vi "位置（目标角度）报文计算公式.vi"(1 "位置":dbl(slide) scale=-12.5..12.5) -> (0 "输出位置报文":string)   [LabVIEW 2023]
panel:
  out "*(类型 *) &x":string
  out "二进制":string
  out "十进制数":i32
  out "位置16进制报文":string
  out "位置转换所得数值":u64
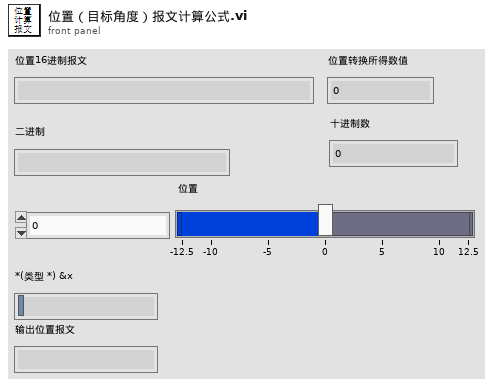
[diagram p1: front panel]
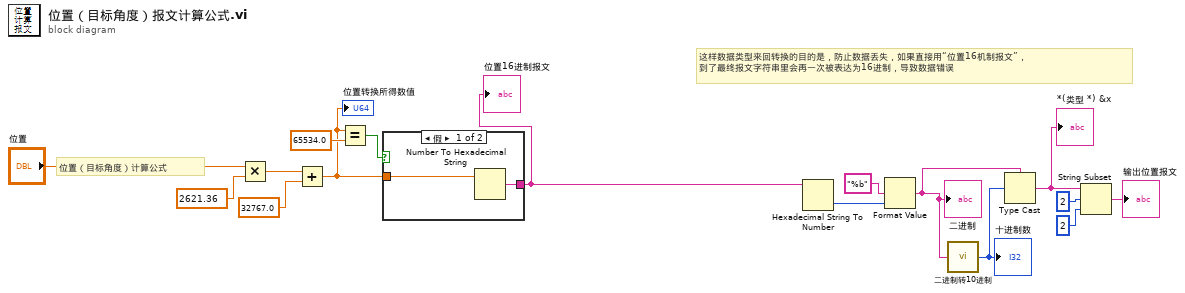
[diagram p0: block diagram]
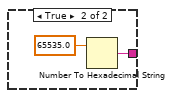
[diagram p2: hidden frame]
diagram:
  # "这样数据类型来回转换的目的是，防止数据丢失，如果直接用“位置16机制报文”，\n到了最终报文字符串里会再一次被表达为16进制，导致数据错误"
  # "位置（目标角度）计算公式"
  n1 = Multiply(x="位置", y=2621.36) -> (x*y=w15:dbl)
  n2 = Add(x=w15, y=32767.0) -> (x+y=w6:dbl)
  "位置转换所得数值" <- w6
  n3 = Equal?(x=w6, y=65534.0) -> (x = y?=w11:bool)
  n4 = case shown="假" w11 {
    tunnel: w6 -> [w17 _]
    tunnel: [w18 w20] -> w5
    frame False {
      n5 = Number To Hexadecimal String(2:w17) -> (0:w18:string)  [unwired: 1 in]
    }
    frame True {
      n6 = Number To Hexadecimal String(2:65535.0) -> (0:w20:string)  [unwired: 1 in]
    }
  }
  "位置16进制报文" <- w5
  n7 = Hexadecimal String To Number(string=w5) -> (number=w9:u32)  [unwired: 2 in, 1 out]
  n8 = Format Value(format string="%b" ("格式字符串"), value (0)=w9) -> (output string=w7:string)  [unwired: 1 in]
  "二进制" <- w7
  n9 = call "二进制转10进制.vi"("字符串"=w7) -> ("十进制数"=w8:i32)
  "十进制数" <- w8
  n10 = Type Cast(type=w7, x=w8) -> (*(type *) &x=w4:string)
  "*(类型 *) &x" <- w4
  n11 = String Subset(string=w4, offset (0)=2 ("偏移量(0)"), length (rest)=2 ("长度（剩余）")) -> (substring=→"输出位置报文":string)
